vi "SG_changePower.vi"(5 "Type":enum16{"Default", "E6680A"}(ring), 7 "dBm":i32, 8 "error in":errorcluster, 11 "VISA in":refnum<visa-resource-name>) -> (0 "error out":errorcluster, 2 "SG_Resp":string, 3 "VISA out":refnum<visa-resource-name>)   [LabVIEW 2023, in "Keysight.lvlib"]
uses:
  Keysight.lvlib
panel:
  in  "Wait(ms)":u32=2000
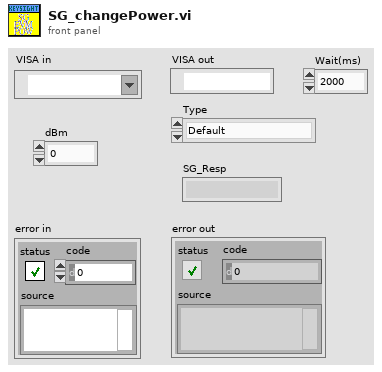
[diagram p1: front panel]
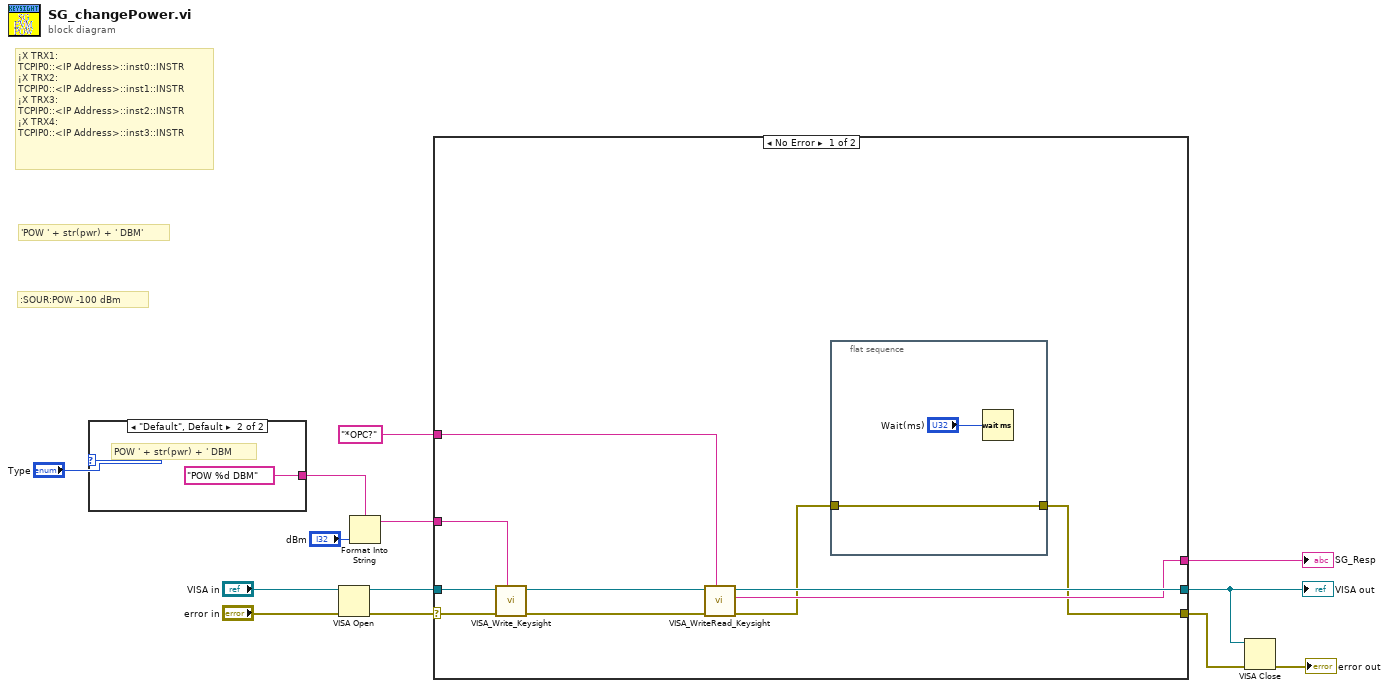
[diagram p0: block diagram]
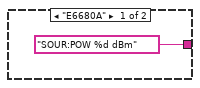
[diagram p2: hidden frame]
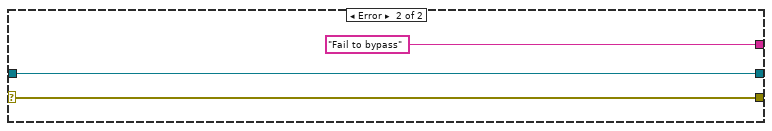
[diagram p3: hidden frame]
diagram:
  # "¡X TRX1:\nTCPIP0::<IP Address>::inst0::INSTR\n¡X TRX2:\nTCPIP0::<IP Address>::inst1::INSTR\n¡X TRX3:\nTCPIP0::<IP Address>::inst2::INSTR\n¡X TRX4:\nTCPIP0::<IP Address>::inst3::INSTR"
  # ":SOUR:POW -100 dBm"
  # "'POW ' + str(pwr) + ' DBM'"
  n1 = case shown="\"Default\", Default" "Type" {
    tunnel: ["SOUR:POW %d dBm" ("format string") "POW %d DBM" ("format string")] -> w11
    frame "E6680A" {
    }
    frame "Default", Default {
      # "POW ' + str(pwr) + ' DBM"
    }
  }
  n2 = VISA Open(error in (no error)="error in", VISA resource name="VISA in") -> (VISA resource name=w6:refnum<visa-resource-name>, error out=w5:errorcluster)  [unwired: 3 in]
  n3 = Format Into String(format string=w11, "dBm") -> (resulting string=w9:string)  [unwired: 2 in, 1 out]
  n4 = case shown="No Error" w5 {
    selector: w5 -> [w25 w29]
    tunnel: w6 -> [w24 w30]
    tunnel: w9 -> [w23 _]
    tunnel: [w16 w29] -> w4
    tunnel: [w22 w30] -> w2
    tunnel: [w21 "Fail to bypass" ("Response")] -> w13
    tunnel: "*OPC?" ("write buffer") -> [w18 _]
    frame No Error {
      n5 = call "VISA_Write_Keysight.vi"("VISA CMD"=w23, "error in"=w25, "VISA in"=w24) -> ("error out"=w19:errorcluster, "VISA out"=w20:refnum<visa-resource-name>)  [unwired: 7 in]
      n6 = call "VISA_WriteRead_Keysight.vi"("VISA_CMD"=w18, "error in"=w19, "VISA in"=w20) -> ("error out"=w17:errorcluster, "Response"=w21:string, "VISA out"=w22:refnum<visa-resource-name>)  [unwired: 6 in]
      n7 = flat-sequence {
        tunnel: w17 -> [w27]
        tunnel: [w27] -> w16
        frame #0 {
          n8 = Wait (ms)(milliseconds to wait="Wait(ms)") -> ()  [unwired: 1 out]
        }
      }
    }
    frame Error {
    }
  }
  "SG_Resp" <- w13
  "VISA out" <- w2
  n9 = VISA Close(VISA resource name=w2, error in (no error)=w4) -> (error out=→"error out":errorcluster)
